vi "Read Display - Form.vi"(8 "error in (no error)":errorcluster, 11 "NT Scalar (Numeric) in":refnum<class "NT Scalar (Numeric).lvclass">) -> (0 "error out":errorcluster, 2 "form":T1, 3 "NT Scalar (Numeric) out":refnum<class "NT Scalar (Numeric).lvclass">)   [LabVIEW 2020, in "PV Access.lvlib" / "PV Data.lvlib" / "NT Scalar (Numeric).lvclass"]
uses:
  NT Scalar (Numeric).lvclass
  1694c7fe-60c7-469f-84c3-0a0c041388b5.vi
  Display Form.ctl
  PV Data.lvlib
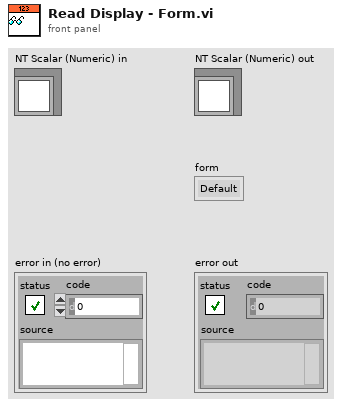
[diagram p1: front panel]
types:
  T1 = typedef "PV Access.lvlib/PV Data.lvlib/Display Form.ctl" = enum16{"Default", "String", "Binary", "Decimal", "Hex", "Exponential", "Engineering"}
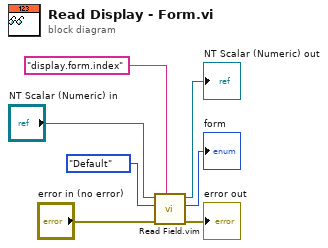
[diagram p0: block diagram]
diagram:
  n1 = call "Read Field.vim"("field"="display.form.index" ("element name"), "error in"="error in (no error)", "default value"=Display_Form."Default" ("Form"), "Base Interface in"="NT Scalar (Numeric) in") -> ("error out"=→"error out":errorcluster, "value"=→"form":T1, "Base Interface out"=→"NT Scalar (Numeric) out":refnum<class "NT Scalar (Numeric).lvclass">)  [unwired: 5 in]
